vi "Cycle Detection.vi"(7 "Stack in":refnum<class "Future.lvclass">[](array[class]), 8 "error in (no error)":errorcluster, 11 "Future in":refnum<class "Future.lvclass">) -> (0 "error out":errorcluster, 1 "Cycle?":bool, 3 "Future out":refnum<class "Future.lvclass">, 5 "Stack out":refnum<class "Future.lvclass">[](array[class]))   [LabVIEW 2017, in "Promise Future.lvlib" / "Future.lvclass"]
uses:
  Future.lvclass
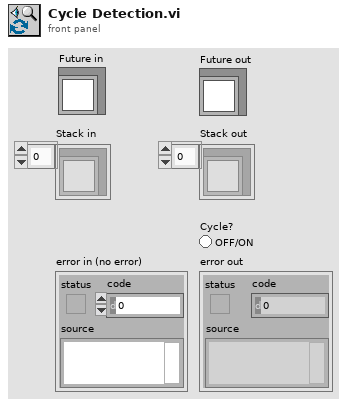
[diagram p1: front panel]
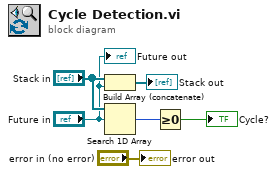
[diagram p0: block diagram]
diagram:
  n1 = Build Array (concatenate)("Stack in", "Future in") -> (→"Stack out":refnum<class "Future.lvclass">[])
  n2 = Search 1D Array(1D array="Stack in", element="Future in") -> (index of element=w2:i32)  [unwired: 1 in]
  n3 = Greater Or Equal To 0?(x=w2) -> (x >= 0?=→"Cycle?":bool)
  "Future out" <- "Future in"
  "error out" <- "error in (no error)"
